vi "JSON to Cluster.vi"(8 "error in":errorcluster, 11 "JSON String":string="{\n    \"firstName\": \"John\",\n    \"lastName\": \"Smith\",\n    \"age\": 25,\n    \"address\": {\n        \"streetAddress\": \"21 2nd Street\",\n        \"city\": \"New York\",\n        \"state\": \"NY\",\n        \"postalCode\": 10021\n    },\n    \"phoneNumbers\": [\n        {\n            \"type\": \"home\",\n            \"number\": \"212 555-1234\"\n        },\n        {\n            \"type\": \"fax\",\n            \"number\": \"646 555-4567\"\n        }\n    ]\n}") -> (0 "error out":errorcluster)   [LabVIEW 2018]
uses:
  <vilib>/Utility/error.llb/Error Cluster From Error Code.vi
  <vilib>/ErrorRing/Error Ring.xnode
panel:
  in  "Simulator Configuration":path=path "C:/Users/celit/Documents/GitHub/client/configurations/simulator.json"
  # "1. Paste JSON string into control and run VI\n2. New VI is created that contains cluster \nrepresentation of the object, and that can\nbe used with the Unflatten from JSON VI"
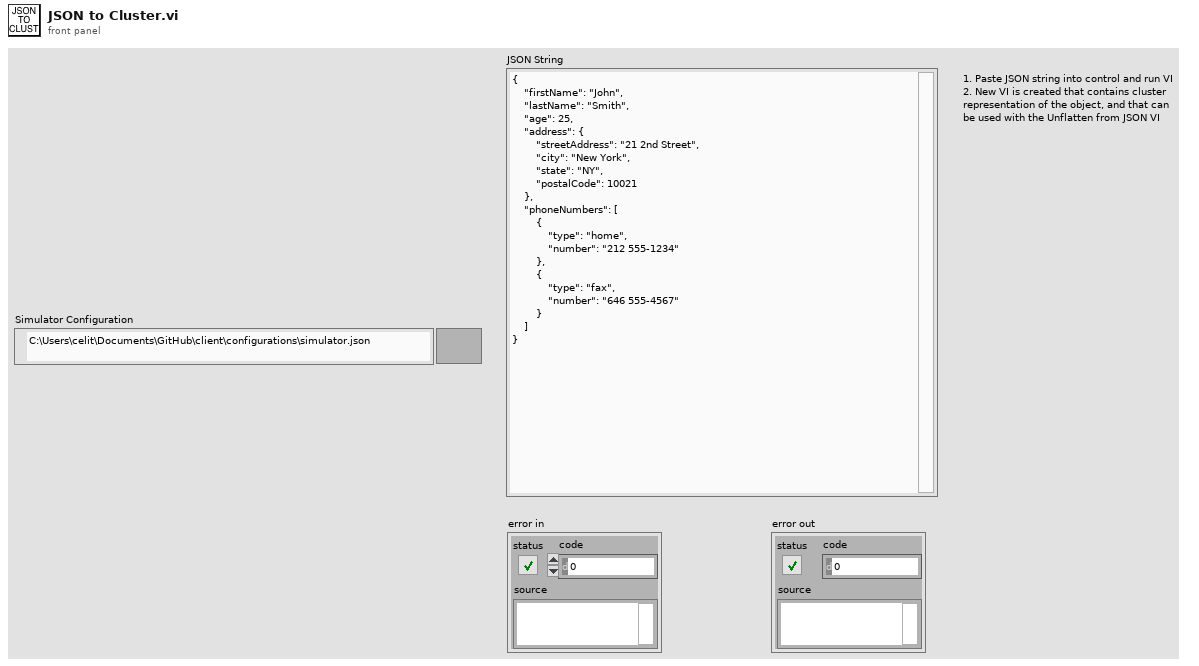
[diagram p1: front panel]
types:
  T1 = typedef "Token.ctl" = enum16{"End", "Boolean", "Named Cluster", "Unnamed Cluster", "Array", "String", "Decimal", "FloatingPoint", "End Array", "End Cluster"}
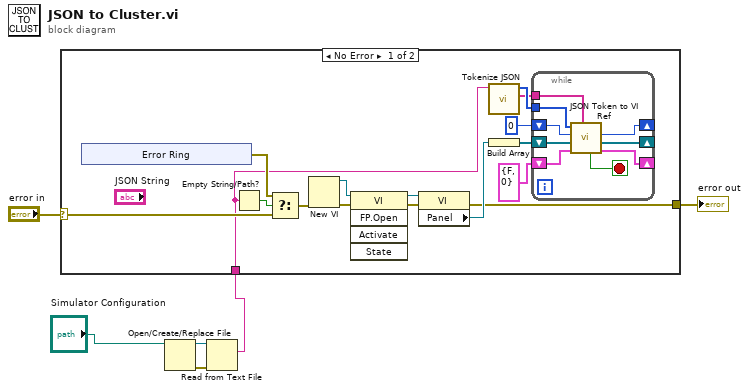
[diagram p0: block diagram]
diagram:
  n1 = Open/Create/Replace File(file path (use dialog)="Simulator Configuration") -> (refnum out=w4:refnum<file>, error out=w3:errorcluster)  [unwired: 5 in, 1 out]
  n2 = Read from Text File(file (use dialog)=w4, error in=w3) -> (text=w1:string)  [unwired: 2 in, 3 out]
  n3 = case shown="No Error" "error in" {
    selector: "error in" -> [w11 w37]
    tunnel: [w8 w37] -> w5
    tunnel: w1 -> [w7 _]
    frame No Error {
      n4 = xnode "Error Ring"() -> ("error out"=w10:errorcluster)
      n5 = Empty String/Path?(string/path=w7) -> (empty?=w12:bool)
      n6 = Select(t=w10, s=w12, f=w11) -> (s? t:f=w9:errorcluster)
      n7 = New VI(8:w9) -> (0:w14:errorcluster, 3:w13:refnum<vi>)  [unwired: 6 in]
      n8 = invoke class="VI" method="FP.Open"(reference=w13, error in=w14) -> (reference out=w19:refnum<vi>, error out=w17:errorcluster)  [unwired: 3 in, 3 out]
      n9 = property class="VI"(reference=w19, error in=w17) -> (error out=w8:errorcluster, "Panel"=w18:refnum<vi>)  [unwired: 1 out]
      n10 = call "Tokenize JSON.vi"("JSON String"=w7) -> ("Variable Names"=w21:string[], "Token Array"=w22:T1[])  [unwired: 9 in]
      n11 = Build Array(w18) -> (w15:refnum<vi>[])
      n12 = while {
        tunnel: w22 -> [w35]
        tunnel: w21 -> [w34]
        shift-right: [w32] -> _
        shift-left: 0 -> [w33]
        shift-right: [w31] -> _
        shift-left: w15 -> [w36]
        shift-right: [w28] -> _
        shift-left: cluster{"In Array?":bool, "Cluster Level":i32} {"In Array?"=FALSE, "Cluster Level"=0} ("Inception Tracking") -> [w29]
        stop <- w30 stop-if-true
        n13 = call "JSON Token to VI Ref.vi"("Variable Names"=w34, "Inception Tracking"=w29, "Parent Ref"=w36, "index"=w33, "Token Array"=w35) -> ("Inception Tracking Out"=w28:cluster{"In Array?":bool, "Cluster Level":i32}, "Parent Ref Out"=w31:refnum<vi>[], "index out"=w32:i32, "End?"=w30:bool)  [unwired: 3 in]
      }
    }
    frame Error {
    }
  }
  "error out" <- w5
